vi "GPIB Write & Read.vi"() -> ()   [LabVIEW 2020]
panel:
  in  "error in":errorcluster
  in  "GPIB Address":i16=1
  in  "Enum":enum16{"Write", "Read", "Write and Read"}(ring)
  in  "milliseconds to wait between write & read":u32
  out "read status":bool[](array[boolean])
  out "String Received":string
  in  "Read mode (0)":i16
  out "error out":errorcluster
  in  "string to send":string
  # "ldu,0,256,8;sdu,0,1024,1024;cl0;omrm;sron"
  # "Status Byte:\n[0]: Dev.Clear State  \n[1]: Dev.Trig.State    \n[2]: Listener Active   \n[3]: Talker Active      \n[4]: Attn. Asserted    \n[5]: CIC                      \n[6]: Remote State       \n[7]: Lockout State      \n[8]: Oper.Complete\n[9]:   ---\n[10]: ---\n[11]: ---\n[12]: SRQ det.whl CIC\n[13]: EOI or EOS det.\n[14]: Timeout\n[15]: Error detected"
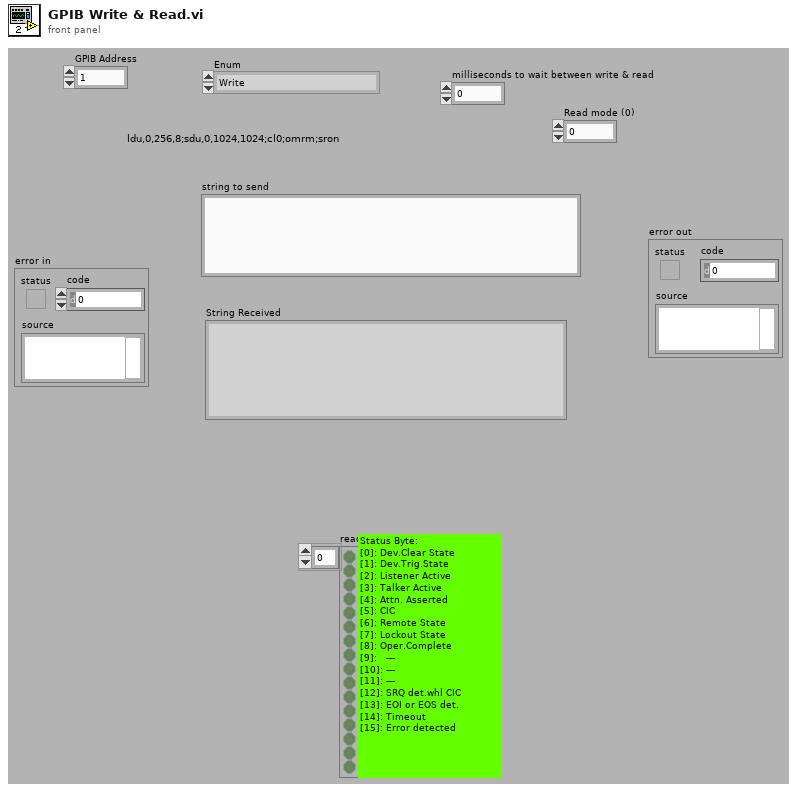
[diagram p1: front panel]
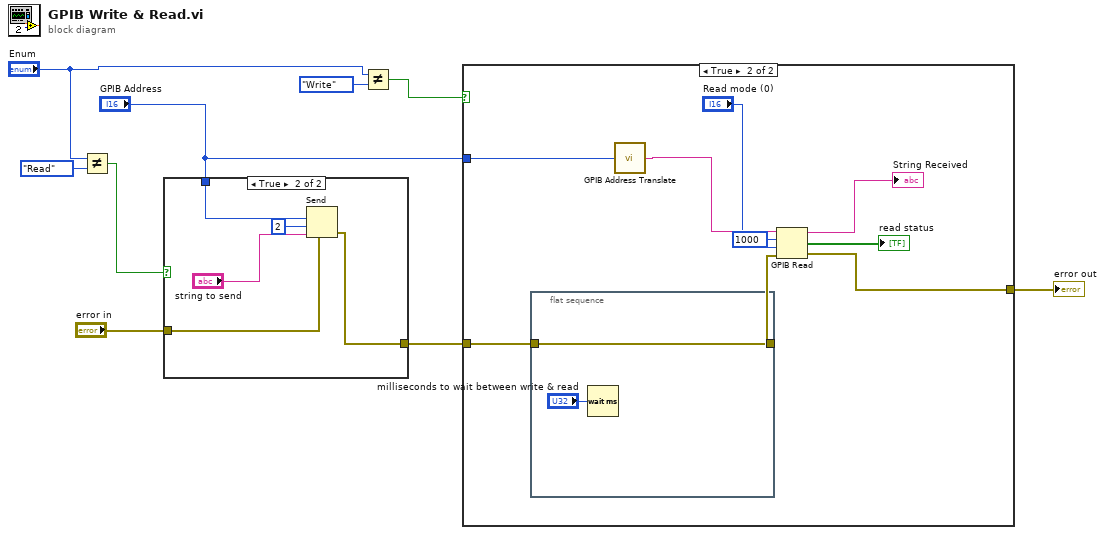
[diagram p0: block diagram]
diagram:
  n1 = Not Equal?(x="Enum", y=enum16{"Write", "Read", "Write and Read"}."Read") -> (x != y?=w6:bool)
  n2 = case shown="True" w6 {
    tunnel: "GPIB Address" -> [_ w13]
    tunnel: [w10 w12] -> w8
    tunnel: "error in" -> [w10 w11]
    frame False {
    }
    frame True {
      n3 = Send(2:w13, 3:i16 2 ("mode"), 4:w11, 5:"string to send") -> (8:w12:errorcluster)  [unwired: 1 in, 2 out]
    }
  }
  n4 = Not Equal?(x="Enum", y=enum16{"Write", "Read", "Write and Read"}."Write") -> (x != y?=w3:bool)
  n5 = case shown="True" w3 {
    tunnel: "GPIB Address" -> [_ w25]
    tunnel: [w16 w20] -> w9
    tunnel: w8 -> [w16 w19]
    frame False {
    }
    frame True {
      n6 = flat-sequence {
        tunnel: [w27] -> w18
        tunnel: w19 -> [w27]
        frame #0 {
          n7 = Wait (ms)(milliseconds to wait="milliseconds to wait between write & read") -> ()  [unwired: 1 out]
        }
      }
      n8 = call "GPIB Address Translate.vi"("GPIB Address"=w25) -> ("GPIB Address String"=w24:string)
      n9 = GPIB Read(0:w24, 1:1000 ("byte count"), 2:"Read mode (0)", 3:w18) -> (5:→"String Received":string, 6:→"read status":bool[], 7:w20:errorcluster)  [unwired: 1 in]
    }
  }
  "error out" <- w9
